vi "sub_strain_balance.vi"(11 "strain_offset_wf":waveform(dbl)[](array[waveform])) -> (2 "Balance":cluster{"X":dbl, "Y":dbl}[](graph), 3 "Balance xy wfs":cluster{"X":dbl, "Y":dbl}[](graph))   [LabVIEW 2016]
uses:
  <vilib>/measure/madcrms.llb/Basic Averaged DC-RMS for 1 Chan.vi
  Global.vi
  <vilib>/measure/NI_MAPro.lvlib
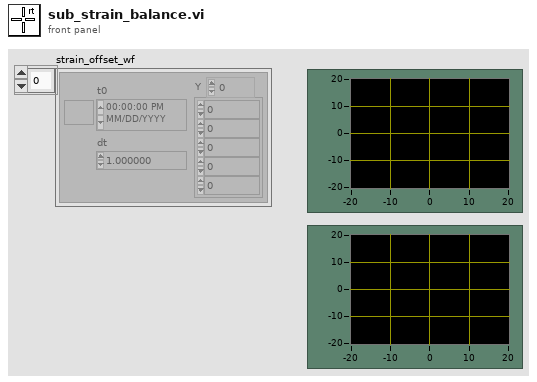
[diagram p1: front panel]
types:
  T1 = typedef "force_sensor_data.ctl" = cluster{"weight":cluster{"front":dbl, "left":dbl, "back":dbl, "right":dbl}, "strain map":cluster{"x":dbl, "y":dbl}[]}
  T2 = cluster{"front":dbl, "left":dbl, "back":dbl, "right":dbl}
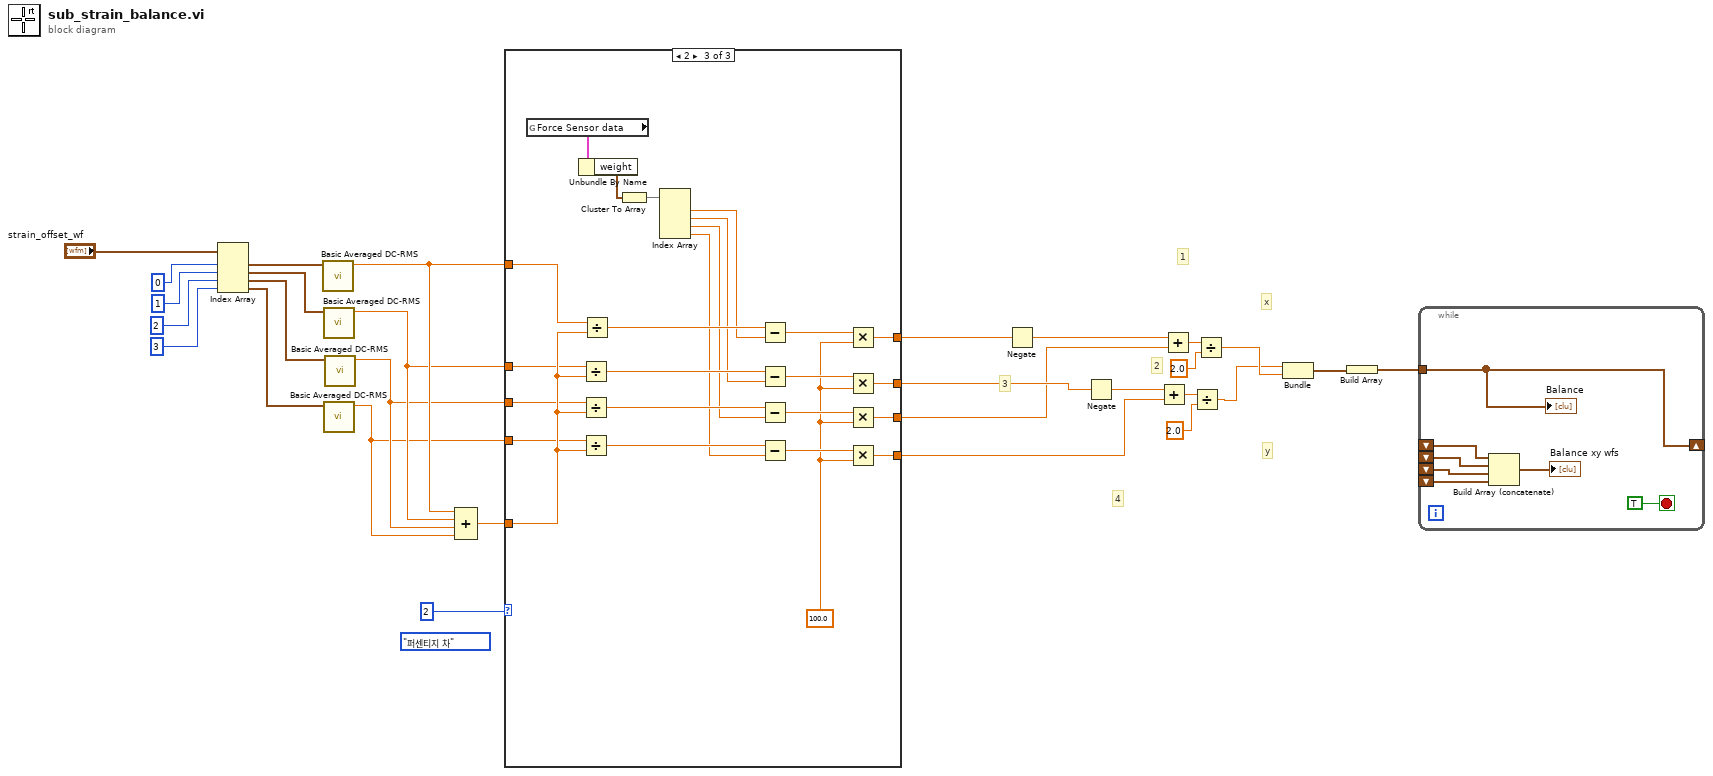
[diagram p0: block diagram]
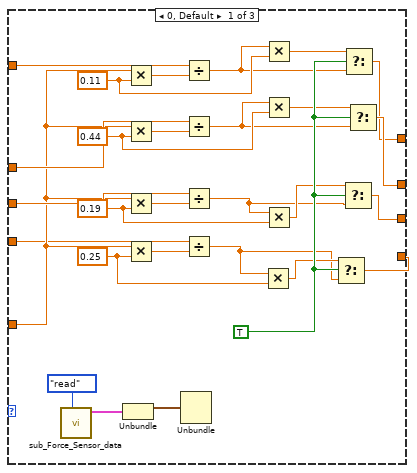
[diagram p2: hidden frame]
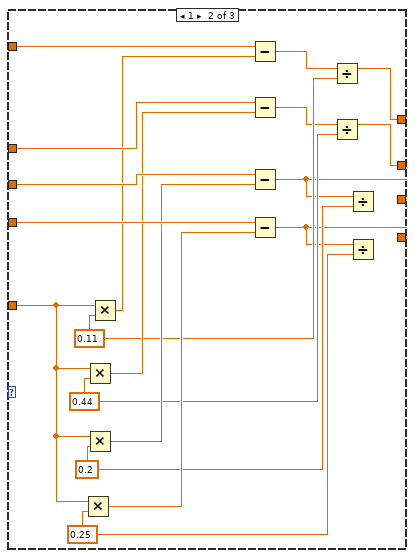
[diagram p3: hidden frame]
diagram:
  (unwired) enum16{"측정-합*비율", "퍼센티지 차"}."퍼센티지 차"
  # "y"
  # "x"
  # "4"
  # "3"
  # "2"
  # "1"
  n1 = Index Array(array="strain_offset_wf", index #1=0, index #2=1, index #3=2, index #4=3) -> (element #1=w17:waveform(dbl), element #2=w16:waveform(dbl), element #3=w15:waveform(dbl), element #4=w14:waveform(dbl))
  n2 = call-poly <vilib>:"Basic Averaged DC-RMS.vi"("signal in"=w17) -> ("DC value"=w22:dbl)  [unwired: 7 in, 3 out]
  n3 = call-poly <vilib>:"Basic Averaged DC-RMS.vi"("signal in"=w16) -> ("DC value"=w21:dbl)  [unwired: 7 in, 3 out]
  n4 = call-poly <vilib>:"Basic Averaged DC-RMS.vi"("signal in"=w14) -> ("DC value"=w19:dbl)  [unwired: 7 in, 3 out]
  n5 = call-poly <vilib>:"Basic Averaged DC-RMS.vi"("signal in"=w15) -> ("DC value"=w20:dbl)  [unwired: 7 in, 3 out]
  n6 = Compound Arithmetic op=ADD(w22, w21, w20, w19) -> (w18:dbl)
  n7 = case shown="2" 2 {
    tunnel: w22 -> [w58 w75 w99]
    tunnel: w21 -> [w55 w74 w98]
    tunnel: w20 -> [w53 w73 w97]
    tunnel: w19 -> [w50 w72 w96]
    tunnel: [w33 w62 w87] -> w4
    tunnel: [w34 w61 w86] -> w3
    tunnel: [w35 w60 w85] -> w2
    tunnel: [w36 w59 w84] -> w1
    tunnel: w18 -> [w51 w67 w100]
    frame 0, Default {
      w45 = TRUE
      w46 = 0.25 ("y")
      w47 = 0.19 ("y")
      w48 = 0.44 ("y")
      w49 = 0.11 ("y")
      n8 = call "sub_Force_Sensor_data.vi"("cmd"=enum16{"write", "read"}."read") -> ("Force Sensor data out"=w31:T1)  [unwired: 10 in]
      n9 = Unbundle(w31) -> ("weight"=w30:T2)  [unwired: 1 out]
      n10 = Multiply(x=w51, y=w49) -> (x*y=w57:dbl)
      n11 = Multiply(x=w51, y=w48) -> (x*y=w56:dbl)
      n12 = Multiply(x=w51, y=w47) -> (x*y=w54:dbl)
      n13 = Multiply(x=w51, y=w46) -> (x*y=w52:dbl)
      n14 = Unbundle(w30) -> ()  [unwired: 4 out]
      n15 = Divide(x=w58, y=w57) -> (x/y=w39:dbl)
      n16 = Divide(x=w55, y=w56) -> (x/y=w40:dbl)
      n17 = Divide(x=w53, y=w54) -> (x/y=w41:dbl)
      n18 = Divide(x=w50, y=w52) -> (x/y=w37:dbl)
      n19 = Multiply(x=w37, y=w46) -> (x*y=w38:dbl)
      n20 = Multiply(x=w39, y=w49) -> (x*y=w44:dbl)
      n21 = Multiply(x=w40, y=w48) -> (x*y=w43:dbl)
      n22 = Multiply(x=w41, y=w47) -> (x*y=w42:dbl)
      n23 = Select(t=w38, s=w45, f=w37) -> (s? t:f=w36:dbl)
      n24 = Select(t=w42, s=w45, f=w41) -> (s? t:f=w35:dbl)
      n25 = Select(t=w44, s=w45, f=w39) -> (s? t:f=w33:dbl)
      n26 = Select(t=w43, s=w45, f=w40) -> (s? t:f=w34:dbl)
    }
    frame 1 {
      w63 = 0.25 ("y")
      w64 = 0.2 ("y")
      w65 = 0.44 ("y")
      w66 = 0.11 ("y")
      n27 = Multiply(x=w67, y=w63) -> (x*y=w68:dbl)
      n28 = Multiply(x=w67, y=w65) -> (x*y=w70:dbl)
      n29 = Multiply(x=w67, y=w64) -> (x*y=w69:dbl)
      n30 = Multiply(x=w67, y=w66) -> (x*y=w71:dbl)
      n31 = Subtract(x=w75, y=w71) -> (x-y=w62:dbl)
      n32 = Subtract(x=w74, y=w70) -> (x-y=w61:dbl)
      n33 = Subtract(x=w73, y=w69) -> (x-y=w60:dbl)
      n34 = Subtract(x=w72, y=w68) -> (x-y=w59:dbl)
      n35 = Divide(x=w62, y=w66) -> ()  [unwired: 1 out]
      n36 = Divide(x=w61, y=w65) -> ()  [unwired: 1 out]
      n37 = Divide(x=w60, y=w64) -> ()  [unwired: 1 out]
      n38 = Divide(x=w59, y=w63) -> ()  [unwired: 1 out]
    }
    frame 2 {
      w76 = 100.0 ("y")
      n39 = global read "Global.vi" "Force Sensor data"() -> (w83:T1)
      n40 = Unbundle By Name(w83) -> ("weight"=w82:T2)
      n41 = Divide(x=w98, y=w100) -> (x/y=w94:dbl)
      n42 = Divide(x=w97, y=w100) -> (x/y=w93:dbl)
      n43 = Divide(x=w96, y=w100) -> (x/y=w92:dbl)
      n44 = Divide(x=w99, y=w100) -> (x/y=w95:dbl)
      n45 = Cluster To Array(cluster=w82) -> (array=w81:dbl[])
      n46 = Index Array(array=w81) -> (element #1=w80:dbl, element #2=w79:dbl, element #3=w78:dbl, element #4=w77:dbl)  [unwired: 4 in]
      n47 = Subtract(x=w95, y=w80) -> (x-y=w91:dbl)
      n48 = Subtract(x=w94, y=w79) -> (x-y=w88:dbl)
      n49 = Subtract(x=w93, y=w78) -> (x-y=w89:dbl)
      n50 = Subtract(x=w92, y=w77) -> (x-y=w90:dbl)
      n51 = Multiply(x=w91, y=w76) -> (x*y=w87:dbl)
      n52 = Multiply(x=w88, y=w76) -> (x*y=w86:dbl)
      n53 = Multiply(x=w89, y=w76) -> (x*y=w85:dbl)
      n54 = Multiply(x=w90, y=w76) -> (x*y=w84:dbl)
    }
  }
  n55 = Negate(x=w4) -> (-x=w28:dbl)
  n56 = Negate(x=w3) -> (-x=w29:dbl)
  n57 = Add(x=w29, y=w1) -> (x+y=w24:dbl)
  n58 = Add(x=w28, y=w2) -> (x+y=w26:dbl)
  n59 = Divide(x=w24, y=2.0) -> (x/y=w7:dbl)
  n60 = Divide(x=w26, y=2.0) -> (x/y=w8:dbl)
  n61 = Bundle(w7, w8) -> (w23:cluster{dbl, dbl})  [unwired: 1 in]
  n62 = Build Array(w23) -> (w6:cluster{dbl, dbl}[])
  n63 = while {
    shift-right: [w106] -> _
    shift-left: _ -> [w102]
    tunnel: w6 -> [w106]
    shift-left: _ -> [w103]
    shift-left: _ -> [w104]
    shift-left: _ -> [w105]
    stop <- TRUE stop-if-true
    n64 = Build Array (concatenate)(w102, w103, w104, w105) -> (→"Balance xy wfs":cluster{dbl, dbl}[])
    "Balance" <- w106
  }
